vi "testgraphtprofile.vi"() -> ()   [LabVIEW 2017]
panel:
  out "Waveform Graph":cluster{dbl, dbl, dbl[][]}(graph)
  out "error out":errorcluster
  in  "error in (no error)":errorcluster
  in  "Path":path=path "C:/Users/stefan/Documents/GitHub/TVAC/head/Labview2017/TVAC_GUI/TestScripts/graphTest.json"
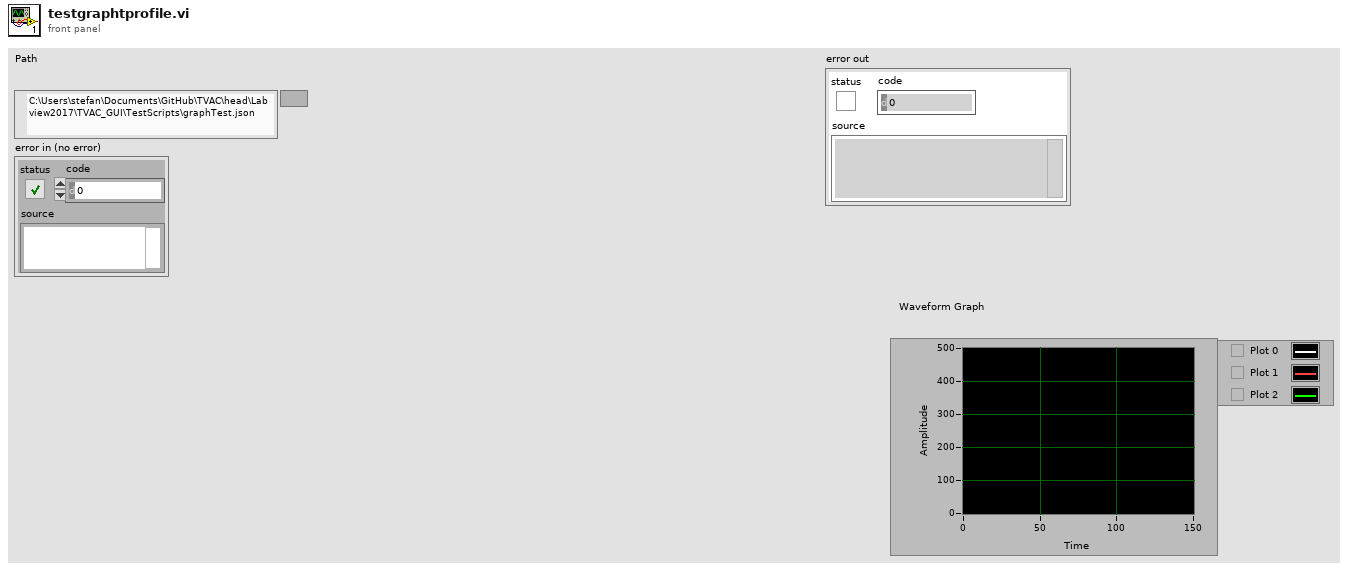
[diagram p1: front panel]
types:
  T1 = cluster{"time":dbl[], "zone1":dbl[], "zone2":dbl[], "zone3":dbl[], "zone4":dbl[], "zone5":dbl[], "zone6":dbl[], "zone7":dbl[], "zone8":dbl[], "zone9":dbl[]}
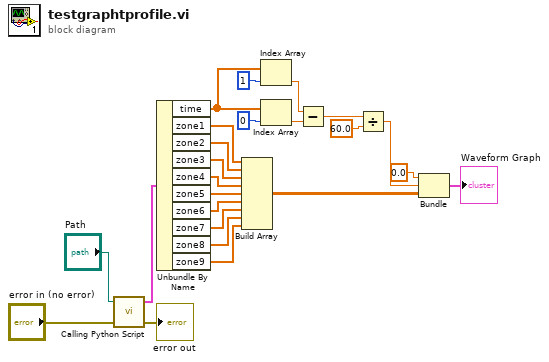
[diagram p0: block diagram]
diagram:
  n1 = call "Calling Python Script.vi"("error in (no error)"="error in (no error)", "Path"="Path") -> ("error out"=→"error out":errorcluster, "graphCluster"=w15:T1)  [unwired: 2 in]
  n2 = Unbundle By Name(w15) -> ("time"=w13:dbl[], "zone1"=w11:dbl[], "zone2"=w10:dbl[], "zone3"=w7:dbl[], "zone4"=w6:dbl[], "zone5"=w5:dbl[], "zone6"=w4:dbl[], "zone7"=w3:dbl[], "zone8"=w2:dbl[], "zone9"=w1:dbl[])
  n3 = Build Array(w11, w10, w7, w6, w5, w4, w3, w2, w1) -> (w17:dbl[][])
  n4 = Index Array(array=w13, index=1) -> (element=w9:dbl)
  n5 = Index Array(array=w13, index=0) -> (element=w8:dbl)
  n6 = Subtract(x=w9, y=w8) -> (x-y=w23:dbl)
  n7 = Divide(x=w23, y=60.0) -> (x/y=w21:dbl)
  n8 = Bundle(0.0, w21, w17) -> (→"Waveform Graph":cluster{dbl, dbl, dbl[][]})  [unwired: 1 in]
